vi "dfd_SOS to TF.vi"(10 "SOS reverse coefficients":dbl[](array[numeric]) format="%.2f", 11 "SOS forward coefficients":dbl[](array[numeric]) format="%.2f") -> (2 "denominator":dbl[](array[numeric]) format="%.2f", 3 "numerator":dbl[](array[numeric]) format="%.2f")   [LabVIEW 2017, in "NI_DigFilterLicensed.lvlib"]
uses:
  <vilib>/addons/Digital Filter Design/NI_DigFilterLicensed.lvlib
  <vilib>/Analysis/2dsp.llb/1D Convolution (DBL).vi
  <vilib>/Analysis/NI_AALPro.lvlib
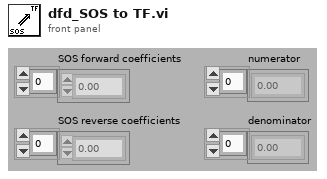
[diagram p1: front panel]
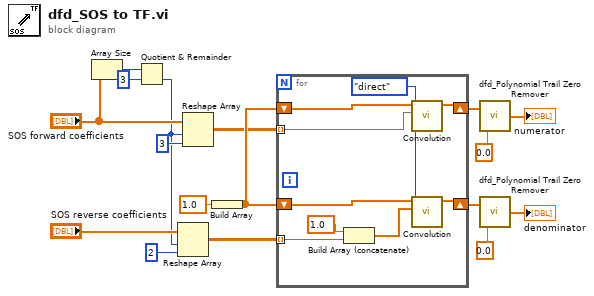
[diagram p0: block diagram]
diagram:
  n1 = Array Size(array="SOS forward coefficients") -> (size(s)=w16:i32)
  n2 = Quotient & Remainder(x=w16, y=3) -> (floor(x/y)=w2:i32)  [unwired: 1 out]
  n3 = Reshape Array("SOS reverse coefficients", w2, 2) -> (w3:dbl[][])
  n4 = Reshape Array("SOS forward coefficients", w2, 3) -> (w5:dbl[][])
  n5 = Build Array(1.0 ("element")) -> (w14:dbl[])
  n6 = for {
    tunnel: w3 -> [w18] mode=indexing
    shift-right: [w24] -> w13
    shift-left: w14 -> [w25]
    shift-right: [w21] -> w11
    shift-left: w14 -> [w22]
    tunnel: w5 -> [w19] mode=indexing
    w20 = enum32{"direct", "frequency domain"}."direct" ("algorithm")
    n7 = Build Array (concatenate)(1.0 ("element"), w18) -> (w23:dbl[])
    n8 = call-poly <vilib>:"Convolution.vi"("algorithm"=w20, "Y"=w19, "X"=w22) -> ("X * Y"=w21:dbl[])  [unwired: 8 out]
    n9 = call-poly <vilib>:"Convolution.vi"("algorithm"=w20, "Y"=w23, "X"=w25) -> ("X * Y"=w24:dbl[])  [unwired: 8 out]
  }
  n10 = call <vilib>:"dfd_Polynomial Trail Zero Remover.vi"("tol"=0.0, "poly in"=w11) -> ("poly out"=→"numerator":dbl[])
  n11 = call <vilib>:"dfd_Polynomial Trail Zero Remover.vi"("tol"=0.0, "poly in"=w13) -> ("poly out"=→"denominator":dbl[])
